vi "Get Python Version.vi"(11 "error in (no error)":errorcluster) -> (2 "Python Version":string, 3 "error out":errorcluster)   [LabVIEW 2021]
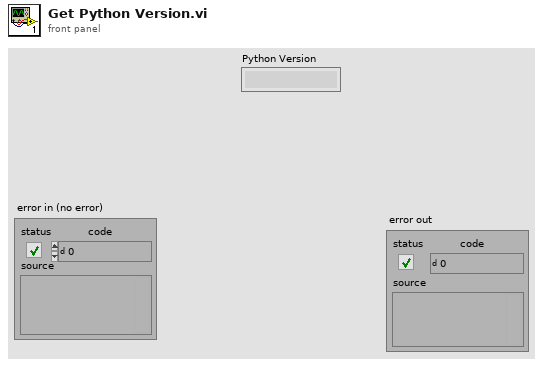
[diagram p1: front panel]
types:
  T1 = typedef "File Paths.ctl" = cluster{"Glue Pattern Folder":path, "Carrier Tray Folder":path, "Pick Up Tool Fixture Folder":path, "Components Folder":path, "Bellows Tool Offset.txt":path, "Pick Up Tool Offset.txt":path, "Dispense Tip Offset.txt":path, "Log Files":path, "Gantry Assembly Map.txt":path, "Syringe and offset map.txt":path, "Controllers Folder":path}
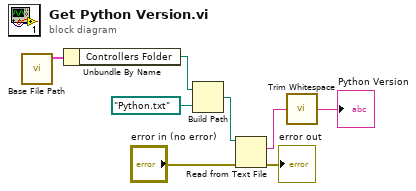
[diagram p0: block diagram]
diagram:
  n1 = call "Base File Path.vi"() -> ("Paths Out"=w7:T1)  [unwired: 11 in]
  n2 = Unbundle By Name(w7) -> ("Controllers Folder"=w6:path)
  n3 = Build Path(base path=w6, name or relative path=path "Python.txt") -> (appended path=w4:path)
  n4 = Read from Text File(file (use dialog)=w4, error in="error in (no error)") -> (text=w3:string, error out=→"error out":errorcluster)  [unwired: 2 in, 2 out]
  n5 = call <vilib>:"Trim Whitespace.vi"("string"=w3) -> ("trimmed string"=→"Python Version":string)  [unwired: 1 in]
